vi "data_inp(2).vi"() -> ()   [LabVIEW 2017]
uses:
  <vilib>/Analysis/baseanly.llb/Mean (DBL).vi
  <instrlib>/Keithley 6517/Keithley 6517.lvlib
  <instrlib>/Lake Shore Cryotronics 332/Lake Shore Cryotronics 332.lvlib
  <vilib>/Analysis/NI_AALBase.lvlib
panel:
  out "error":i32
  out "mean":dbl format="%0.2f"
  in  "milliseconds to wait 2":u32
  out "mean array":dbl[][](array[numeric])
  out "XY Graph":cluster{dbl[], dbl[]}(graph)
  out "appended array":dbl[][](array[numeric])
  in  "number of readings":i32
  out "Kelvin Reading":dbl min=0.0 max=1645.0 step=1e-05 format="%^.5e"
  in  "Lakeshore":refnum<visa-resource-name>
  out "Measurement 3":dbl
  in  "Keithley":refnum<visa-resource-name>
  out "Keithley_out":refnum<visa-resource-name>
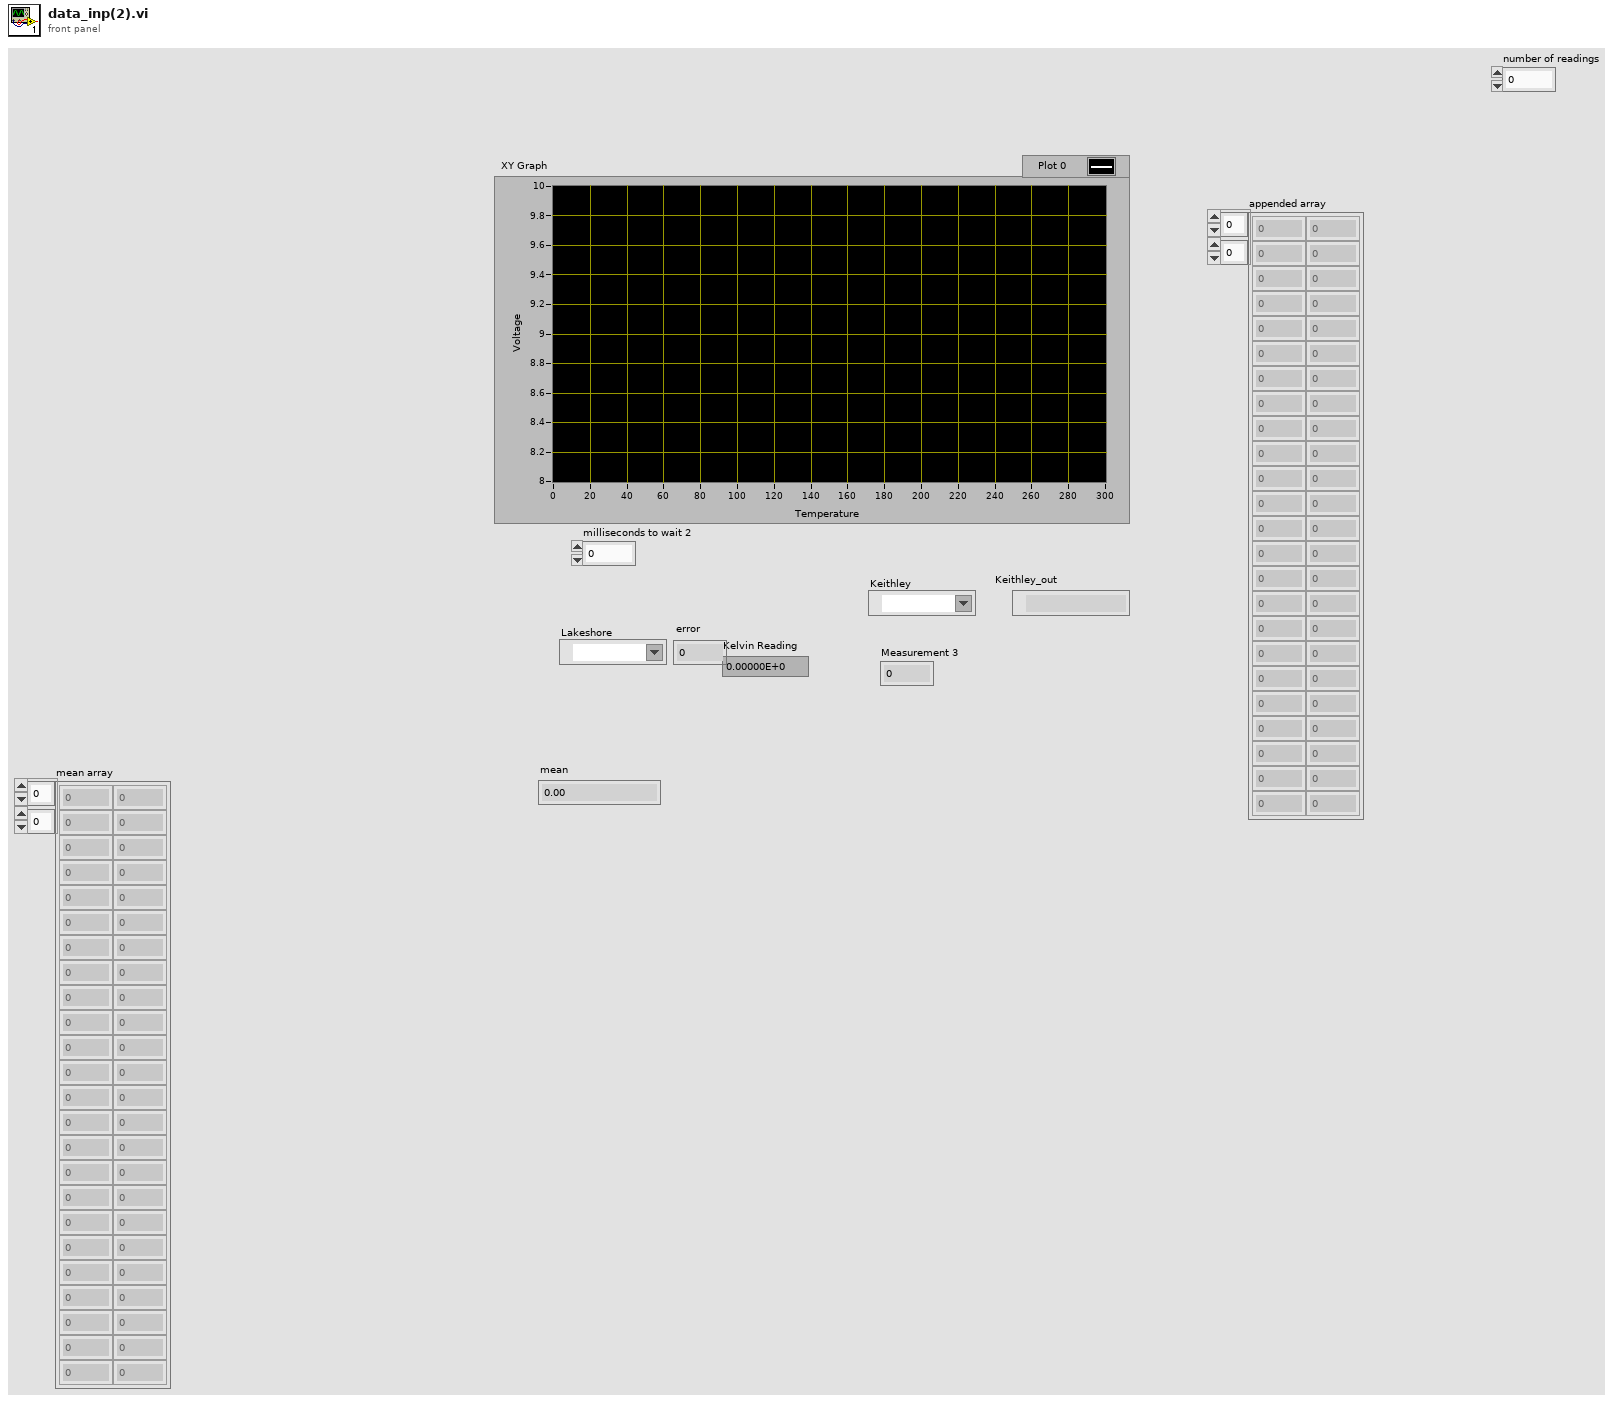
[diagram p1: front panel]
types:
  T1 = cluster{"Measurement":dbl, "Units":string, "Time Stamp and Date":string, "Reading #":dbl, "Channel #":dbl}
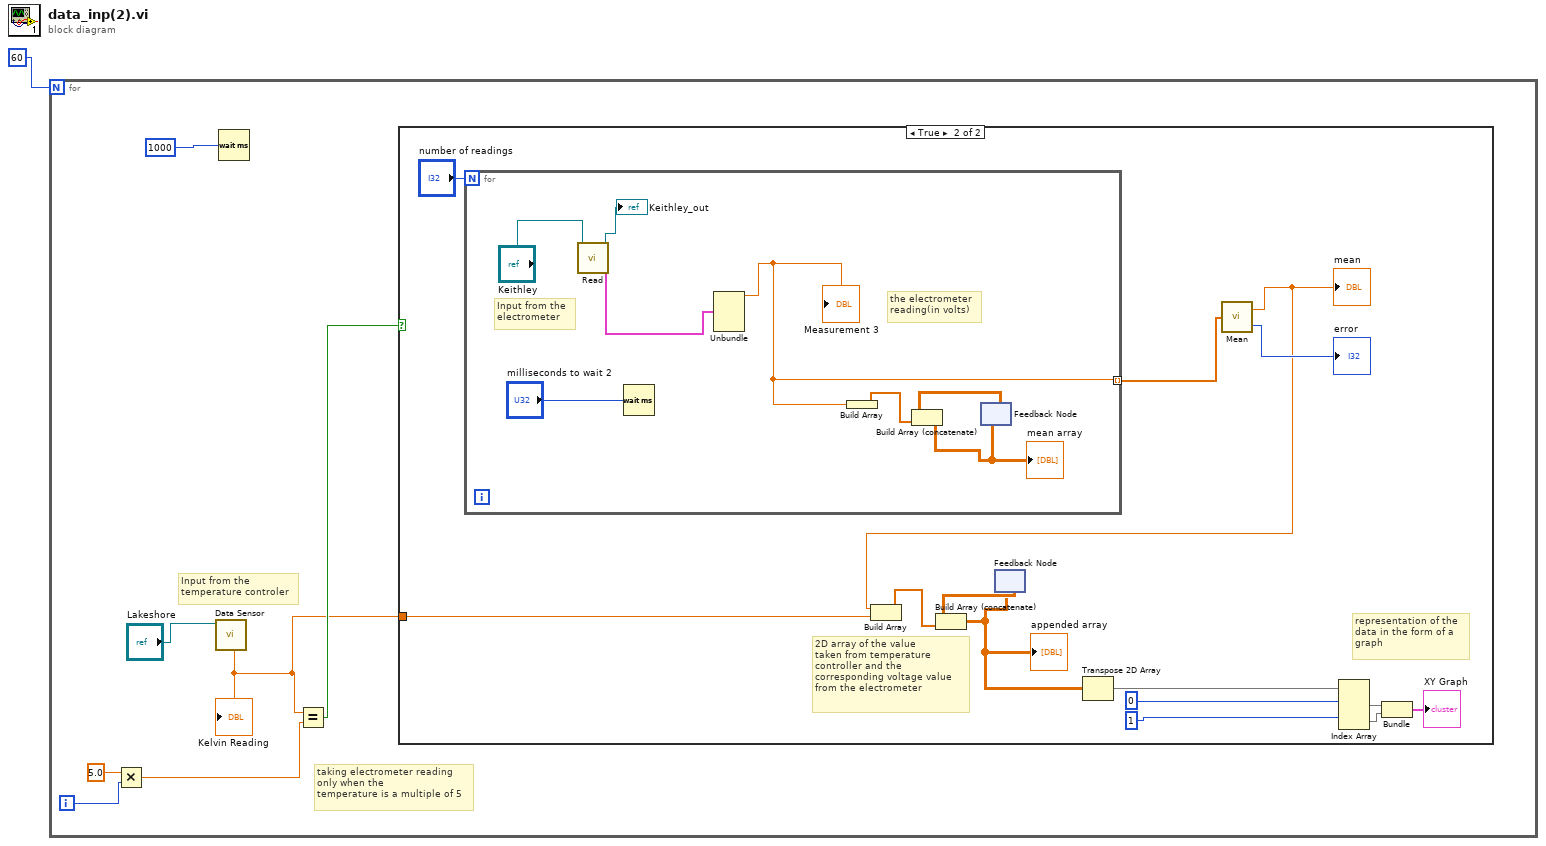
[diagram p0: block diagram]
diagram:
  n1 = for {
    N: 60 -> [_]
    i -> [w7]
    # "taking electrometer reading\nonly when the \ntemperature is a multiple of 5"
    # "Input from the \ntemperature controler"
    n2 = Multiply(x=5.0, y=w7) -> (x*y=w5:dbl)
    n3 = call <instrlib>:"Data Sensor.vi"("VISA resource name"="Lakeshore") -> ("Kelvin Reading"=w3:dbl)  [unwired: 6 in, 4 out]
    "Kelvin Reading" <- w3
    n4 = Wait (ms)(milliseconds to wait=u32 1000) -> ()  [unwired: 1 out]
    n5 = Equal?(x=w3, y=w5) -> (x = y?=w4:bool)
    n6 = case shown="True" w4 {
      tunnel: w3 -> [_ w12]
      frame False {
      }
      frame True {
        # "representation of the \ndata in the form of a\ngraph"
        # "2D array of the value\ntaken from temperature\ncontroller and the\ncorresponding voltage value \nfrom the electrometer"
        n7 = for {
          N: "number of readings" -> [_]
          tunnel: [w23] -> w10 mode=indexing
          # "the electrometer \nreading(in volts)"
          # "Input from the\nelectrometer"
          n8 = call <instrlib>:"Read.vi"("VISA resource name"="Keithley") -> ("Measurement"=w28:T1, "VISA resource name out"=→"Keithley_out":refnum<visa-resource-name>)  [unwired: 8 in, 1 out]
          n9 = Wait (ms)(milliseconds to wait="milliseconds to wait 2") -> ()  [unwired: 1 out]
          n10 = Unbundle(w28) -> ("Measurement"=w23:dbl)  [unwired: 4 out]
          "Measurement 3" <- w23
          n11 = Build Array(w23) -> (w27:dbl[])
          n12 = feedback #1() -> (w26:dbl[][])  [unwired: 1 in]
          n13 = Build Array (concatenate)(w26, w27) -> (w24:dbl[][])
          "mean array" <- w24
          n14 = feedback-in #1(w24) -> ()
        }
        n15 = feedback #2() -> (w20:dbl[][])  [unwired: 1 in]
        n16 = call-poly <vilib>:"Mean.vi"("X"=w10) -> ("mean"=w9:dbl, "error"=→"error":i32)
        "mean" <- w9
        n17 = Build Array(w9, w12) -> (w21:dbl[])
        n18 = Build Array (concatenate)(w20, w21) -> (w13:dbl[][])
        "appended array" <- w13
        n19 = feedback-in #2(w13) -> ()
        n20 = Transpose 2D Array(2D array=w13) -> (transposed array=w14:dbl[][])
        n21 = Index Array(array=w14, index (row) #1=0 ("index (row)"), index (row) #2=1 ("index (row)")) -> (element #1=w17:dbl[], element #2=w16:dbl[])  [unwired: 2 in]
        n22 = Bundle(w17, w16) -> (→"XY Graph":cluster{dbl[], dbl[]})  [unwired: 1 in]
      }
    }
  }
